vi "AddSpaces.vi"(7 "Text.Selection":T1, 8 "Add Spaces?":bool, 11 "String in":refnum<vi>) -> (1 "Cursor":cluster{u32, u32}, 3 "String out":refnum<vi>)   [LabVIEW 2016, in "Code.xctl"]
uses:
  <userlib>/MicroPython/VIs/ColorText/Code.xctl
  <vilib>/Utility/miscctls.llb/LVSelectionTypeDef.ctl
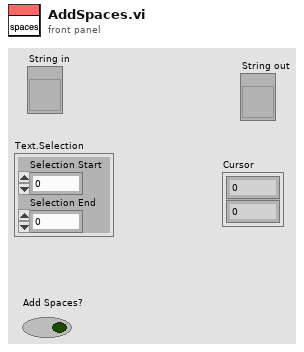
[diagram p1: front panel]
types:
  T1 = typedef "LVSelectionTypeDef.ctl" = cluster{"Selection Start":u32, "Selection End":u32}
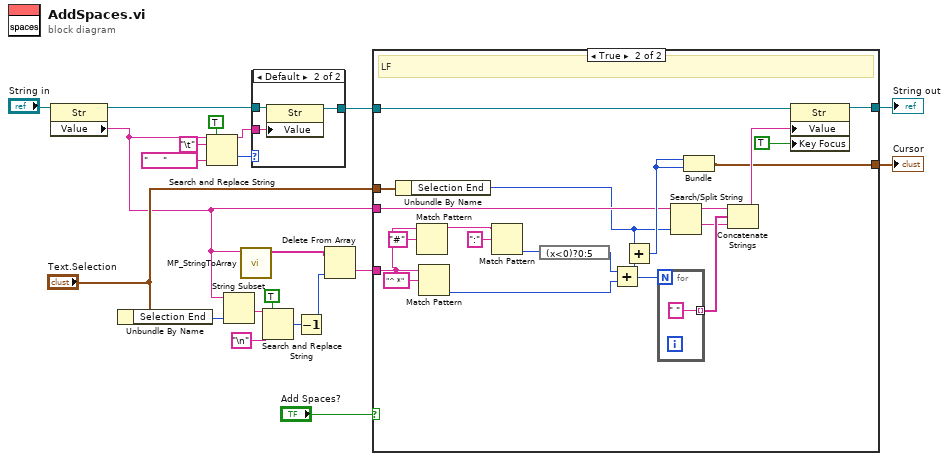
[diagram p0: block diagram]
diagram:
  n1 = property on="Property Node" class="Str"(reference="String in") -> (reference out=w2:refnum<vi>, "Value"=w1:string)  [unwired: 1 in, 1 out]
  n2 = Unbundle By Name("Text.Selection") -> ("Selection End"=w17:u32)
  n3 = Search and Replace String(replace all?=TRUE ("replace all? (F)"), input string=w1, search string="\t", replace string="     " ("replace string (\"\")")) -> (result string=w5:string, number of replacements=w6:i32)  [unwired: 4 in, 2 out]
  n4 = String Subset(string=w1, length (rest)=w17) -> (substring=w16:string)  [unwired: 1 in]
  n5 = call <userlib>:"MP_StringToArray.vi"("write buffer"=w1) -> ("Array"=w11:string[])  [unwired: 10 in]
  n6 = case shown="Default" w6 {
    tunnel: w2 -> [w22 w25]
    tunnel: [w22 w24] -> w4
    tunnel: w5 -> [_ w23]
    frame 0 {
    }
    frame Default {
      n7 = property on="Property Node" class="Str"(reference=w25, "Value"=w23) -> (reference out=w24:refnum<vi>)  [unwired: 1 in, 1 out]
    }
  }
  n8 = Search and Replace String(replace all?=TRUE ("replace all? (F)"), input string=w16, search string="\n") -> (number of replacements=w13:i32)  [unwired: 5 in, 3 out]
  n9 = Decrement(x=w13) -> (x-1=w12:i32)
  n10 = Delete From Array(array=w11, index=w12) -> (deleted portion=w21:string)  [unwired: 1 in, 1 out]
  n11 = case shown="True" "Add Spaces?" {
    tunnel: w21 -> [_ w47]
    tunnel: w1 -> [_ w32]
    tunnel: w4 -> [w26 w39]
    tunnel: [w26 w38] -> w20
    tunnel: "Text.Selection" -> [w27 w35]
    tunnel: [w27 w28] -> w10
    frame False {
    }
    frame True {
      # "LF"
      n12 = Unbundle By Name(w35) -> ("Selection End"=w31:u32)
      n13 = Match Pattern(string=w47, regular expression="#") -> (before substring=w44:string)  [unwired: 1 in, 3 out]
      n14 = Match Pattern(string=w47, regular expression="^ *") -> (offset past match=w41:i32)  [unwired: 1 in, 3 out]
      n15 = Match Pattern(string=w44, regular expression=":") -> (offset past match=w43:i32)  [unwired: 1 in, 3 out]
      n16 = expression code="(x<0)?0:5"(w43) -> (w42:i32)
      n17 = Add(x=w42, y=w41) -> (x+y=w34:i32)
      n18 = Add(x=w31, y=w34) -> (x+y=w33:u32)
      n19 = for {
        N: w34 -> [_]
        tunnel: [" " ("regular expression")] -> w40 mode=indexing
      }
      n20 = Search/Split String(string=w32, offset (0)=w31) -> (substring before match=w30:string, match + rest of string=w29:string)  [unwired: 1 in, 1 out]
      n21 = Bundle(w33, w33) -> (w28:cluster{u32, u32})  [unwired: 1 in]
      n22 = Concatenate Strings(w30, w40, w29) -> (w37:string)
      n23 = property class="Str"(reference=w39, "Value"=w37, "Key Focus"=TRUE) -> (reference out=w38:refnum<vi>)  [unwired: 1 in, 1 out]
    }
  }
  "String out" <- w20
  "Cursor" <- w10
